vi "PID_controller_19.vi"() -> ()   [LabVIEW 2011]
panel:
  out "Angle (deg)":dbl format="%.1f"
  in  "Local":bool
  in  "Hold":bool
  out "tune_Method":u16(ring) items=["Setpoint", "Angle"]
  in  "Method":u16(ring)=1 items=["Setpoint", "Angle"]
  in  "Setpoint":u16(ring)=2 items=["A", "B", "C", "D"]
  out "do_tune":bool
  in  "Tune":bool
  out "Tune Set Point (torr)":dbl format="%.2f"
  in  "stop":bool
  out "fit":cluster{"element":dbl, "Value":dbl}[](array[cluster])
  out "err_avg":dbl
  out "Setpoint":string
  in  "Ks":dbl
  out "dt(s)":dbl
  out "windup error":dbl
  out "tPrev":dbl
  out "target value":dbl
  out "error(t-t0)":cluster{dbl, "Value":dbl}[](array[cluster])
  out "error":dbl
  out "tStart(s)":dbl
  out "S00":dbl
  out "S10":dbl
  out "S20":dbl
  out "S11":dbl
  out "S01":dbl
  out "weight":dbl[](array[numeric])
  in  "# of points to watch":i32=60
  in  "tSmooth(s)":dbl=4.0
  out "t0":dbl
  out "error(t)":cluster{dbl, "Value":dbl}[](array[cluster])
  out "IO error":errorcluster
  out "first":bool=TRUE
  out "XY Graph":T1(graph)
  out "current value":dbl
  in  "Period (s)":dbl=1.0
  out "dValue":dbl
  out "derivative":dbl
  out "integral":dbl
  in  "Angle (deg)":dbl format="%.1f"
  in  "Kd":dbl=0.4
  in  "Ki":dbl
  in  "Kp":dbl=0.1
  out "P (torr)":dbl format="%.2f"
  in  "Set Point (torr)":dbl format="%.2f"
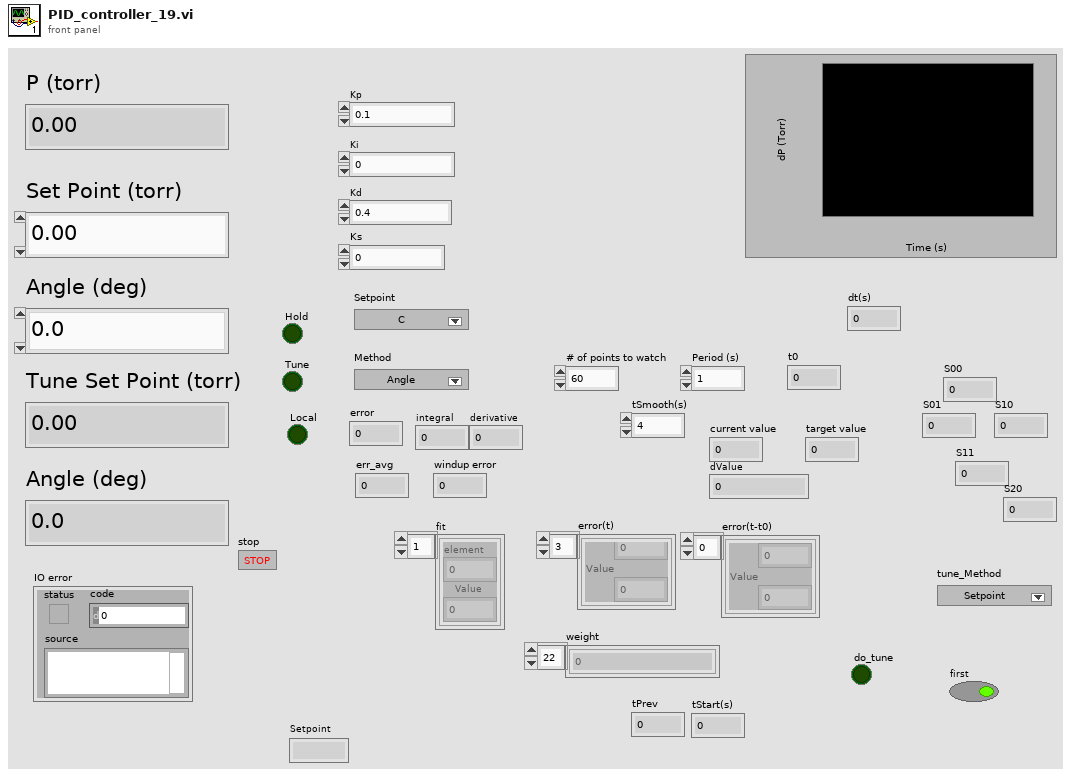
[diagram p1: front panel]
types:
  T1 = cluster{"Value":cluster{"element":dbl, "Value":dbl}[]}[]
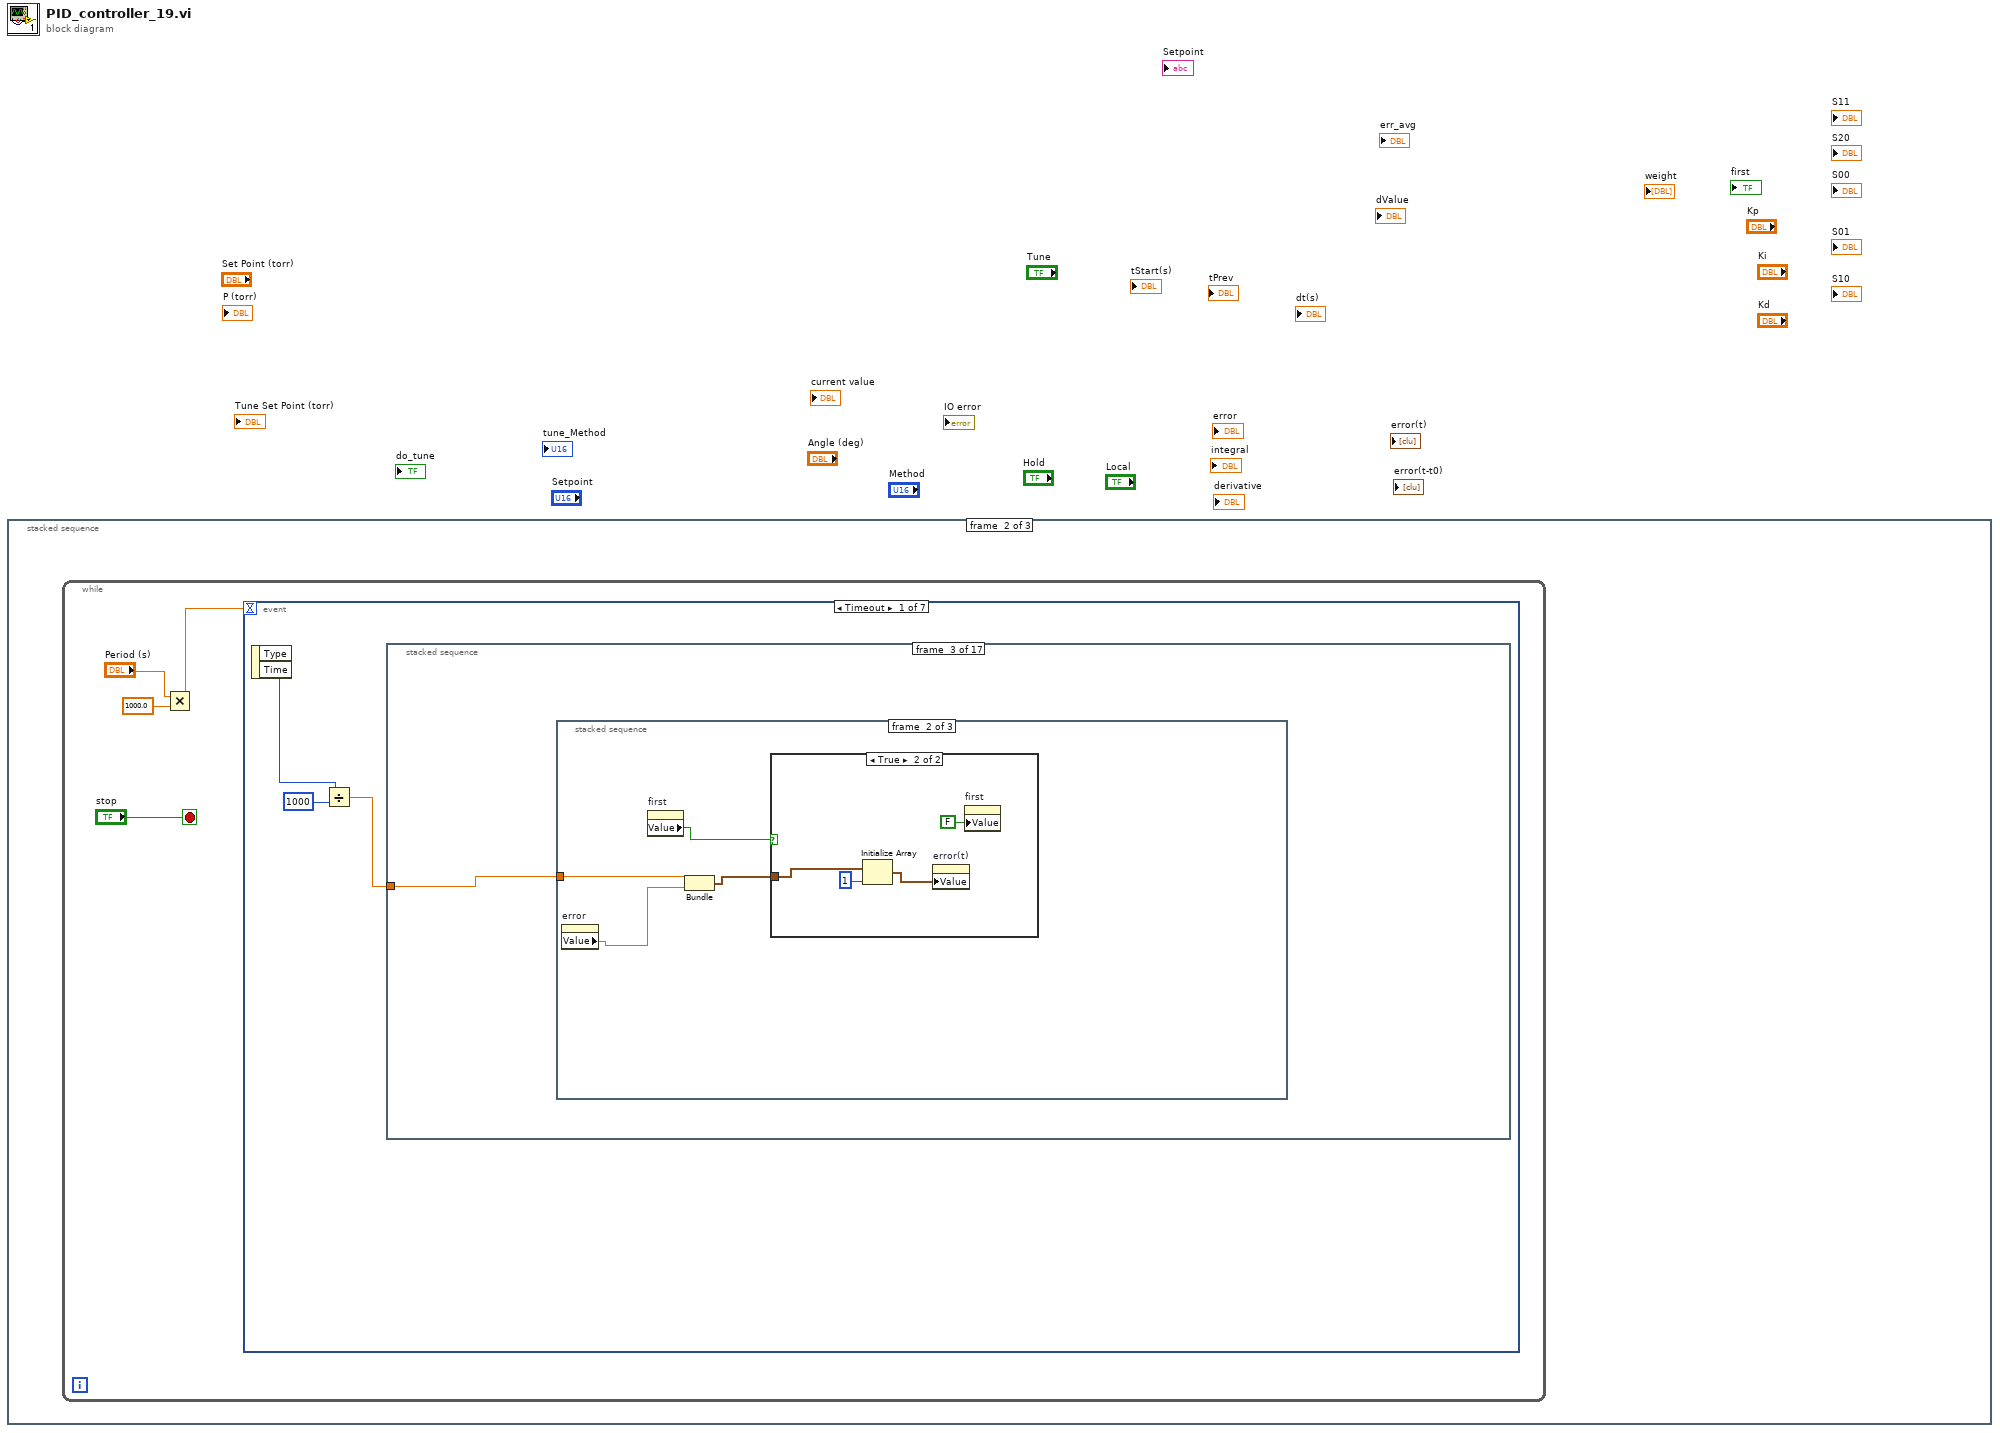
[diagram p0: block diagram]
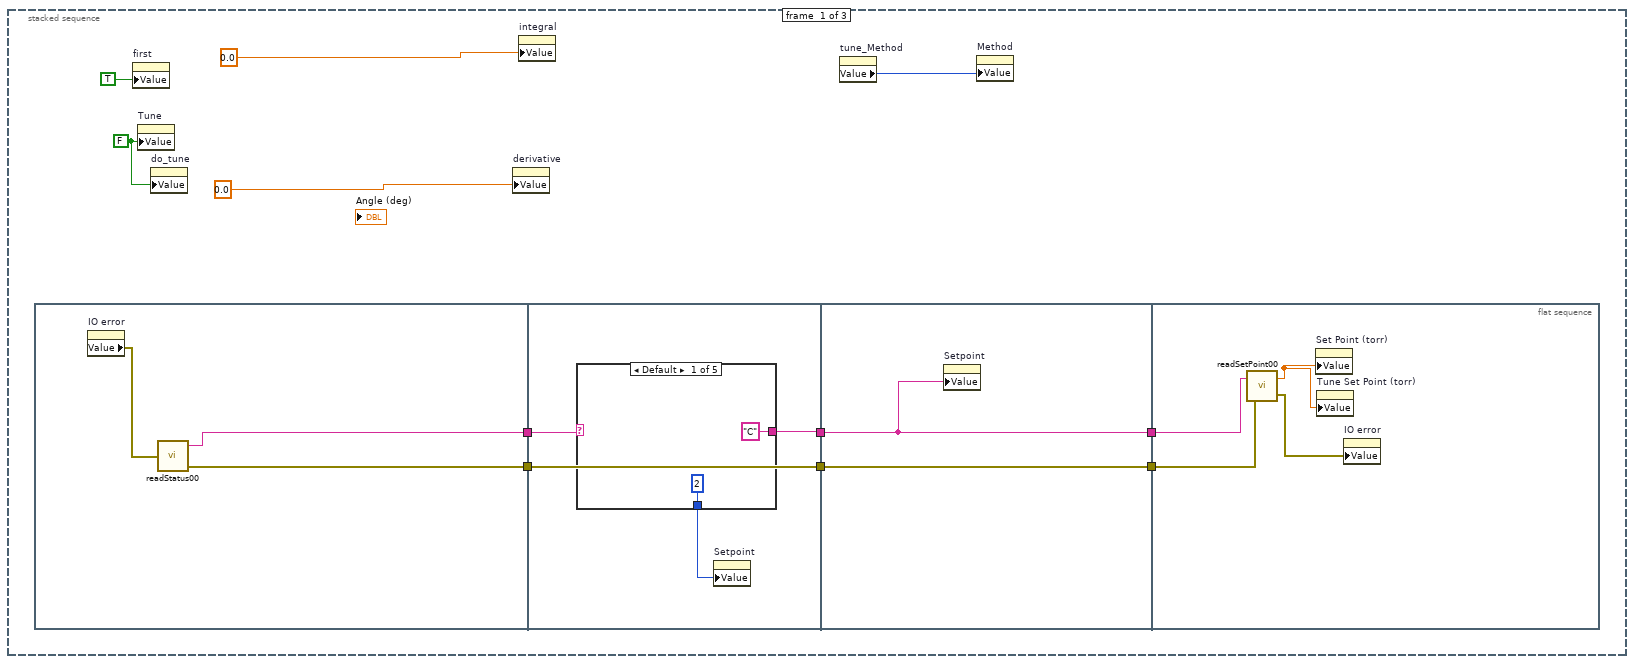
[diagram p2: hidden frame]
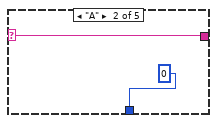
[diagram p3: hidden frame]
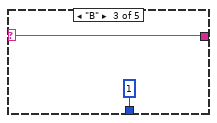
[diagram p4: hidden frame]
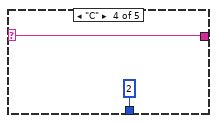
[diagram p5: hidden frame]
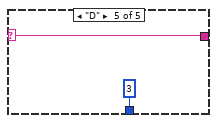
[diagram p6: hidden frame]
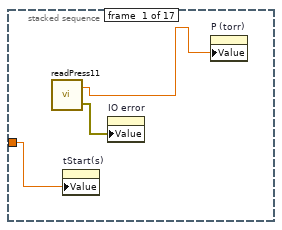
[diagram p7: hidden frame]
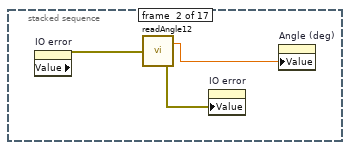
[diagram p8: hidden frame]
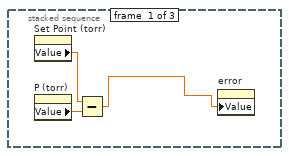
[diagram p9: hidden frame]
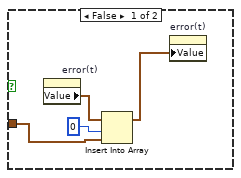
[diagram p10: hidden frame]
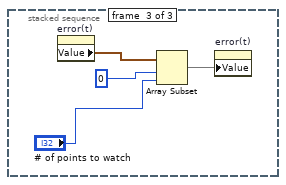
[diagram p11: hidden frame]
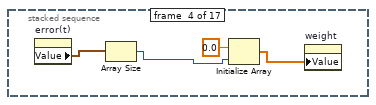
[diagram p12: hidden frame]
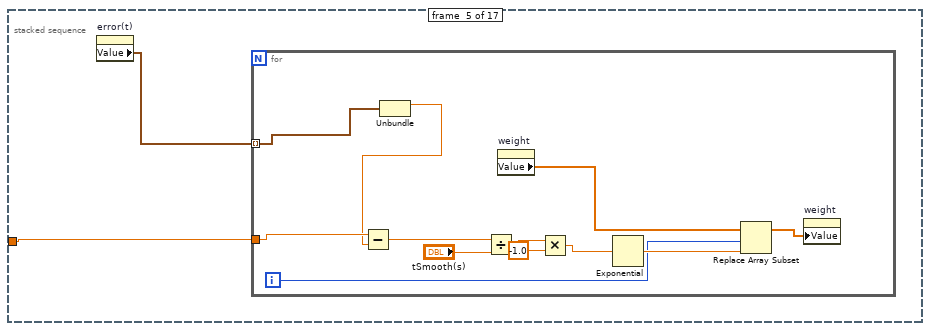
[diagram p13: hidden frame]
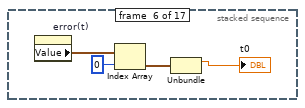
[diagram p14: hidden frame]
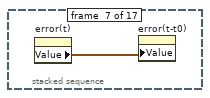
[diagram p15: hidden frame]
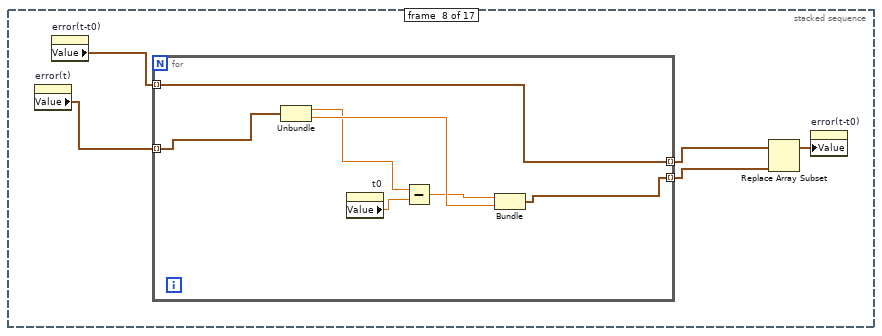
[diagram p16: hidden frame]
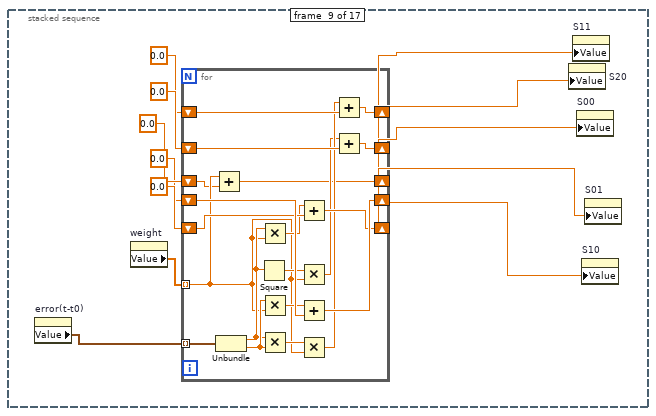
[diagram p17: hidden frame]
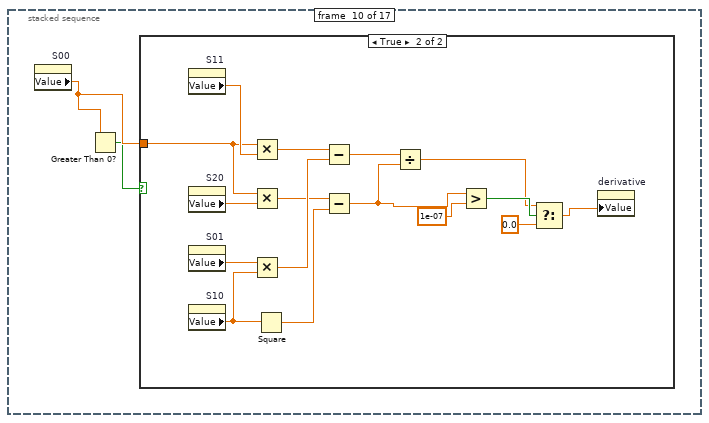
[diagram p18: hidden frame]
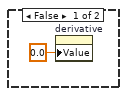
[diagram p19: hidden frame]
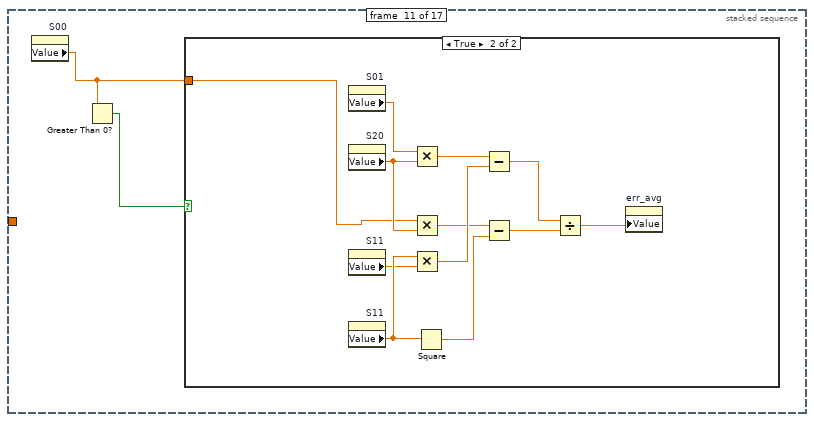
[diagram p20: hidden frame]
diagram:
  n1 = stacked-sequence {
    frame #0 {
      w8 = FALSE ("Tune")
      n2 = flat-sequence {
        tunnel: [w13] -> w7
        tunnel: [w12] -> w6
        tunnel: w7 -> [w17]
        tunnel: [w16] -> w5
        tunnel: w6 -> [w18]
        tunnel: [w18] -> w3
        tunnel: w5 -> [w29]
        tunnel: [w29] -> w4
        tunnel: w3 -> [w30]
        tunnel: [w30] -> w2
        tunnel: w4 -> [w34]
        tunnel: w2 -> [w33]
        frame #0 {
          n3 = property on="IO error" class="Clust (strict)"() -> ("Value"=w14:errorcluster)  [unwired: 2 in, 2 out]
          n4 = call "readStatus00.vi"("error in"=w14) -> ("Setpoint"=w13:string, "error out"=w12:errorcluster)  [unwired: 1 out]
        }
        frame #1 {
          n5 = case shown="Default" w17 {
            selector: w17 -> [_ w22 w23 w25 w27]
            tunnel: ["C" w22 w23 w25 w27] -> w16
            tunnel: [u16 2 ("Ring") u16 0 ("Ring") u16 1 ("Ring") u16 2 ("Ring") u16 3 ("Ring")] -> w15
            frame Default {
            }
            frame "A" {
            }
            frame "B" {
            }
            frame "C" {
            }
            frame "D" {
            }
          }
          n6 = property on="Setpoint" class="Ring (strict)"("Value"=w15) -> ()  [unwired: 2 in, 2 out]
        }
        frame #2 {
          n7 = property on="Setpoint" class="Str"("Value"=w29) -> ()  [unwired: 2 in, 2 out]
        }
        frame #3 {
          n8 = call "readSetPoint00.vi"("error in"=w33, "Setpoint"=w34) -> ("error out"=w32:errorcluster, "P"=w31:dbl)
          n9 = property on="Set Point (torr)" class="DigNum (strict)"("Value"=w31) -> ()  [unwired: 2 in, 2 out]
          n10 = property on="Tune Set Point (torr)" class="DigNum (strict)"("Value"=w31) -> ()  [unwired: 2 in, 2 out]
          n11 = property on="IO error" class="Clust (strict)"("Value"=w32) -> ()  [unwired: 2 in, 2 out]
        }
      }
      n12 = property on="first" class="Bool (strict)"("Value"=TRUE ("first")) -> ()  [unwired: 2 in, 2 out]
      n13 = property on="Tune" class="Bool (strict)"("Value"=w8) -> ()  [unwired: 2 in, 2 out]
      n14 = property on="do_tune" class="Bool (strict)"("Value"=w8) -> ()  [unwired: 2 in, 2 out]
      n15 = property on="derivative" class="DigNum (strict)"("Value"=0.0 ("derivative")) -> ()  [unwired: 2 in, 2 out]
      n16 = property on="integral" class="DigNum (strict)"("Value"=0.0 ("integral")) -> ()  [unwired: 2 in, 2 out]
      n17 = property on="tune_Method" class="Ring (strict)"() -> ("Value"=w1:u16)  [unwired: 2 in, 2 out]
      n18 = property on="Method" class="Ring (strict)"("Value"=w1) -> ()  [unwired: 2 in, 2 out]
    }
    frame #1 {
      n19 = while {
        stop <- "stop" stop-if-true
        n20 = Multiply(x="Period (s)", y=1000.0) -> (x*y=w36:dbl)
        n21 = event shown="[0] Timeout" {
          selector: _ -> [_ _ _ _ _ _ _]
          dyn-events: _ -> [_ _ _ _ _ _ _]
          timeout: w36 -> [_ _ _ _ _ _ _]
          event Timeout {
            n22 = event-data() -> ("Time"=w41:u32)  [unwired: 1 in, 1 out]
            n23 = Divide(x=w41, y=u32 1000) -> (x/y=w39:dbl)
            n24 = stacked-sequence {
              tunnel: w39 -> [w42 _ w48 _ w72 _ _ _ _ _ _ _ _ _ _ _ _]
              frame #0 {
                n25 = call "readPress11.vi"() -> ("P"=w44:dbl, "error out"=w43:errorcluster)  [unwired: 1 in]
                n26 = property on="tStart(s)" class="DigNum (strict)"("Value"=w42) -> ()  [unwired: 2 in, 2 out]
                n27 = property on="IO error" class="Clust (strict)"("Value"=w43) -> ()  [unwired: 2 in, 2 out]
                n28 = property on="P (torr)" class="DigNum (strict)"("Value"=w44) -> ()  [unwired: 2 in, 2 out]
              }
              frame #1 {
                n29 = property on="IO error" class="Clust (strict)"() -> ("Value"=w46:errorcluster)  [unwired: 2 in, 2 out]
                n30 = call "readAngle12.vi"("error in"=w46) -> ("angle"=w47:dbl, "error out"=w45:errorcluster)
                n31 = property on="IO error" class="Clust (strict)"("Value"=w45) -> ()  [unwired: 2 in, 2 out]
                n32 = property on="Angle (deg)" class="DigNum (strict)"("Value"=w47) -> ()  [unwired: 2 in, 2 out]
              }
              frame #2 {
                n33 = stacked-sequence {
                  tunnel: w48 -> [_ w54 _]
                  frame #0 {
                    n34 = property on="Set Point (torr)" class="DigNum (strict)"() -> ("Value"=w50:dbl)  [unwired: 2 in, 2 out]
                    n35 = property on="P (torr)" class="DigNum (strict)"() -> ("Value"=w51:dbl)  [unwired: 2 in, 2 out]
                    n36 = Subtract(x=w50, y=w51) -> (x-y=w49:dbl)
                    n37 = property on="error" class="DigNum (strict)"("Value"=w49) -> ()  [unwired: 2 in, 2 out]
                  }
                  frame #1 {
                    n38 = property on="error" class="DigNum (strict)"() -> ("Value"=w52:dbl)  [unwired: 2 in, 2 out]
                    n39 = property on="first" class="Bool (strict)"() -> ("Value"=w55:bool)  [unwired: 2 in, 2 out]
                    n40 = Bundle(w54, "Value"=w52) -> (w53:cluster{dbl, "Value":dbl})  [unwired: 1 in]
                    n41 = case shown="True" w55 {
                      tunnel: w53 -> [w57 w62]
                      frame False {
                        n42 = property on="error(t)" class="Arr (strict)"() -> ("Value"=w58:cluster{dbl, "Value":dbl}[])  [unwired: 2 in, 2 out]
                        n43 = Insert Into Array(array=w58, index=0, new element=w57) -> (w56:cluster{dbl, "Value":dbl}[])
                        n44 = property on="error(t)" class="Arr (strict)"("Value"=w56) -> ()  [unwired: 2 in, 2 out]
                      }
                      frame True {
                        n45 = Initialize Array(w62, 1 ("dimension size")) -> (w60:cluster{dbl, "Value":dbl}[])
                        n46 = property on="error(t)" class="Arr (strict)"("Value"=w60) -> ()  [unwired: 2 in, 2 out]
                        n47 = property on="first" class="Bool (strict)"("Value"=FALSE ("first")) -> ()  [unwired: 2 in, 2 out]
                      }
                    }
                  }
                  frame #2 {
                    n48 = property on="error(t)" class="Arr (strict)"() -> ("Value"=w65:cluster{dbl, "Value":dbl}[])  [unwired: 2 in, 2 out]
                    n49 = Array Subset(array=w65, index=0, length="# of points to watch") -> (w67:cluster{dbl, "Value":dbl}[])
                    n50 = property on="error(t)" class="Arr (strict)"("Value"=w67) -> ()  [unwired: 2 in, 2 out]
                  }
                }
              }
              frame #3 {
                n51 = property on="error(t)" class="Arr (strict)"() -> ("Value"=w68:cluster{dbl, "Value":dbl}[])  [unwired: 2 in, 2 out]
                n52 = Array Size(array=w68) -> (size(s)=w70:i32)
                n53 = Initialize Array(0.0 ("element"), w70) -> (w71:dbl[])
                n54 = property on="weight" class="Arr (strict)"("Value"=w71) -> ()  [unwired: 2 in, 2 out]
              }
              frame #4 {
                n55 = property on="error(t)" class="Arr (strict)"() -> ("Value"=w73:cluster{dbl, "Value":dbl}[])  [unwired: 2 in, 2 out]
                n56 = for {
                  tunnel: w73 -> [w85] mode=indexing
                  tunnel: w72 -> [w84]
                  i -> [w80]
                  n57 = Unbundle(w85) -> (w83:dbl)  [unwired: 1 out]
                  n58 = Subtract(x=w84, y=w83) -> (x-y=w78:dbl)
                  n59 = Divide(x=w78, y="tSmooth(s)") -> (x/y=w76:dbl)
                  n60 = property on="weight" class="Arr (strict)"() -> ("Value"=w81:dbl[])  [unwired: 2 in, 2 out]
                  n61 = Multiply(x=w76, y=-1.0) -> (x*y=w74:dbl)
                  n62 = Exponential(1:w74) -> (0:w82:dbl)
                  n63 = Replace Array Subset(array=w81, new element=w82, index=w80) -> (w79:dbl[])
                  n64 = property on="weight" class="Arr (strict)"("Value"=w79) -> ()  [unwired: 2 in, 2 out]
                }
              }
              frame #5 {
                n65 = property on="error(t)" class="Arr (strict)"() -> ("Value"=w86:cluster{dbl, "Value":dbl}[])  [unwired: 2 in, 2 out]
                n66 = Index Array(array=w86, index=0) -> (element=w88:cluster{dbl, "Value":dbl})
                n67 = Unbundle(w88) -> (→"t0":dbl)  [unwired: 1 out]
              }
              frame #6 {
                n68 = property on="error(t)" class="Arr (strict)"() -> ("Value"=w90:cluster{dbl, "Value":dbl}[])  [unwired: 2 in, 2 out]
                n69 = property on="error(t-t0)" class="Arr (strict)"("Value"=w90) -> ()  [unwired: 2 in, 2 out]
              }
              frame #7 {
                n70 = property on="error(t)" class="Arr (strict)"() -> ("Value"=w91:cluster{dbl, "Value":dbl}[])  [unwired: 2 in, 2 out]
                n71 = property on="error(t-t0)" class="Arr (strict)"() -> ("Value"=w93:cluster{dbl, "Value":dbl}[])  [unwired: 2 in, 2 out]
                n72 = for {
                  tunnel: w91 -> [w98] mode=indexing
                  tunnel: [w97] -> w92 mode=indexing
                  tunnel: w93 -> [w96] mode=indexing
                  tunnel: [w96] -> w94 mode=indexing
                  n73 = Unbundle(w98) -> (w99:dbl, "Value"=w101:dbl)
                  n74 = property on="t0" class="DigNum (strict)"() -> ("Value"=w102:dbl)  [unwired: 2 in, 2 out]
                  n75 = Subtract(x=w99, y=w102) -> (x-y=w100:dbl)
                  n76 = Bundle(w100, "Value"=w101) -> (w97:cluster{dbl, "Value":dbl})  [unwired: 1 in]
                }
                n77 = Replace Array Subset(array=w94, new element=w92) -> (w95:cluster{dbl, "Value":dbl}[])  [unwired: 1 in]
                n78 = property on="error(t-t0)" class="Arr (strict)"("Value"=w95) -> ()  [unwired: 2 in, 2 out]
              }
              frame #8 {
                n79 = property on="error(t-t0)" class="Arr (strict)"() -> ("Value"=w114:cluster{dbl, "Value":dbl}[])  [unwired: 2 in, 2 out]
                n80 = property on="weight" class="Arr (strict)"() -> ("Value"=w107:dbl[])  [unwired: 2 in, 2 out]
                n81 = for {
                  tunnel: w114 -> [w130] mode=indexing
                  shift-right: [w131] -> w112
                  shift-left: 0.0 -> [w134]
                  shift-right: [w127] -> w109
                  shift-left: 0.0 -> [w133]
                  shift-right: [w126] -> w110
                  shift-left: 0.0 -> [w132]
                  shift-right: [w128] -> w113
                  shift-left: 0.0 -> [w129]
                  tunnel: w107 -> [w117] mode=indexing
                  shift-right: [w115] -> w111
                  shift-left: 0.0 -> [w116]
                  n82 = Add(x=w117, y=w116) -> (x+y=w115:dbl)
                  n83 = Unbundle(w130) -> (w119:dbl, "Value"=w125:dbl)
                  n84 = Square(x=w119) -> (x^2=w121:dbl)
                  n85 = Multiply(x=w119, y=w117) -> (x*y=w118:dbl)
                  n86 = Multiply(x=w125, y=w117) -> (x*y=w124:dbl)
                  n87 = Multiply(x=w119, y=w125) -> (x*y=w123:dbl)
                  n88 = Add(x=w118, y=w129) -> (x+y=w128:dbl)
                  n89 = Multiply(x=w121, y=w117) -> (x*y=w120:dbl)
                  n90 = Add(x=w124, y=w134) -> (x+y=w131:dbl)
                  n91 = Multiply(x=w123, y=w117) -> (x*y=w122:dbl)
                  n92 = Add(x=w122, y=w133) -> (x+y=w127:dbl)
                  n93 = Add(x=w120, y=w132) -> (x+y=w126:dbl)
                }
                n94 = property on="S20" class="DigNum (strict)"("Value"=w110) -> ()  [unwired: 2 in, 2 out]
                n95 = property on="S11" class="DigNum (strict)"("Value"=w109) -> ()  [unwired: 2 in, 2 out]
                n96 = property on="S00" class="DigNum (strict)"("Value"=w111) -> ()  [unwired: 2 in, 2 out]
                n97 = property on="S10" class="DigNum (strict)"("Value"=w113) -> ()  [unwired: 2 in, 2 out]
                n98 = property on="S01" class="DigNum (strict)"("Value"=w112) -> ()  [unwired: 2 in, 2 out]
              }
              frame #9 {
                n99 = property on="S00" class="DigNum (strict)"() -> ("Value"=w136:dbl)  [unwired: 2 in, 2 out]
                n100 = Greater Than 0?(x=w136) -> (x > 0?=w135:bool)
                n101 = case shown="True" w135 {
                  tunnel: w136 -> [_ w145]
                  frame False {
                    n102 = property on="derivative" class="DigNum (strict)"("Value"=0.0 ("derivative")) -> ()  [unwired: 2 in, 2 out]
                  }
                  frame True {
                    n103 = property on="S11" class="DigNum (strict)"() -> ("Value"=w147:dbl)  [unwired: 2 in, 2 out]
                    n104 = property on="S20" class="DigNum (strict)"() -> ("Value"=w146:dbl)  [unwired: 2 in, 2 out]
                    n105 = property on="S01" class="DigNum (strict)"() -> ("Value"=w144:dbl)  [unwired: 2 in, 2 out]
                    n106 = property on="S10" class="DigNum (strict)"() -> ("Value"=w148:dbl)  [unwired: 2 in, 2 out]
                    n107 = Multiply(x=w145, y=w147) -> (x*y=w153:dbl)
                    n108 = Multiply(x=w145, y=w146) -> (x*y=w151:dbl)
                    n109 = Multiply(x=w144, y=w148) -> (x*y=w152:dbl)
                    n110 = Square(x=w148) -> (x^2=w150:dbl)
                    n111 = Subtract(x=w153, y=w152) -> (x-y=w149:dbl)
                    n112 = Subtract(x=w151, y=w150) -> (x-y=w143:dbl)
                    n113 = Divide(x=w149, y=w143) -> (x/y=w139:dbl)
                    n114 = Greater?(x=w143, y=1e-07) -> (0:w141:bool)
                    n115 = Select(t=w139, s=w141, f=0.0) -> (s? t:f=w140:dbl)
                    n116 = property on="derivative" class="DigNum (strict)"("Value"=w140) -> ()  [unwired: 2 in, 2 out]
                  }
                }
              }
              frame #10 {
                n117 = property on="S00" class="DigNum (strict)"() -> ("Value"=w155:dbl)  [unwired: 2 in, 2 out]
                n118 = Greater Than 0?(x=w155) -> (x > 0?=w154:bool)
                n119 = case shown="True" w154 {
                  tunnel: w155 -> [_ w158]
                  frame False {
                    n120 = property on="err_avg" class="DigNum (strict)"("Value"=0.0 ("Pavg")) -> ()  [unwired: 2 in, 2 out]
                  }
                  frame True {
                    n121 = property on="S01" class="DigNum (strict)"() -> ("Value"=w159:dbl)  [unwired: 2 in, 2 out]
                    n122 = property on="S20" class="DigNum (strict)"() -> ("Value"=w162:dbl)  [unwired: 2 in, 2 out]
                    n123 = property on="S11" class="DigNum (strict)"() -> ("Value"=w160:dbl)  [unwired: 2 in, 2 out]
                    n124 = property on="S11" class="DigNum (strict)"() -> ("Value"=w161:dbl)  [unwired: 2 in, 2 out]
                    n125 = Multiply(x=w159, y=w162) -> (x*y=w167:dbl)
                    n126 = Multiply(x=w158, y=w162) -> (x*y=w164:dbl)
                    n127 = Multiply(x=w161, y=w160) -> (x*y=w168:dbl)
                    n128 = Square(x=w161) -> (x^2=w165:dbl)
                    n129 = Subtract(x=w167, y=w168) -> (x-y=w163:dbl)
                    n130 = Subtract(x=w164, y=w165) -> (x-y=w166:dbl)
                    n131 = Divide(x=w163, y=w166) -> (x/y=w157:dbl)
                    n132 = property on="err_avg" class="DigNum (strict)"("Value"=w157) -> ()  [unwired: 2 in, 2 out]
                  }
                }
              }
              frame #11 {
                n133 = property on="error(t-t0)" class="Arr (strict)"() -> ("Value"=w169:cluster{dbl, "Value":dbl}[])  [unwired: 2 in, 2 out]
                n134 = Array Size(array=w169) -> (size(s)=w170:i32)
                n135 = Greater?(x=w170, y=1) -> (0:w172:bool)
                n136 = case shown="True" w172 {
                  frame False {
                  }
                  frame True {
                    n137 = property on="error(t-t0)" class="Arr (strict)"() -> ("Value"=w184:cluster{dbl, "Value":dbl}[])  [unwired: 2 in, 2 out]
                    n138 = Array Size(array=w184) -> (size(s)=w192:i32)
                    n139 = Index Array(array=w184, index=0) -> (element=w190:cluster{dbl, "Value":dbl})
                    n140 = property on="tSmooth(s)" class="DigNum (strict)"() -> ("Value"=w174:dbl)  [unwired: 2 in, 2 out]
                    n141 = Unbundle(w190) -> (w180:dbl)  [unwired: 1 out]
                    n142 = Decrement(x=w192) -> (x-1=w191:i32)
                    n143 = Index Array(array=w184, index=w191) -> (element=w189:cluster{dbl, "Value":dbl})
                    n144 = Multiply(x=w174, y=2.0) -> (x*y=w173:dbl)
                    n145 = Unbundle(w189) -> (w179:dbl)  [unwired: 1 out]
                    n146 = Subtract(x=w180, y=w173) -> (x-y=w177:dbl)
                    n147 = Greater?(x=w179, y=w177) -> (0:w178:bool)
                    n148 = property on="derivative" class="DigNum (strict)"() -> ("Value"=w188:dbl)  [unwired: 2 in, 2 out]
                    n149 = Select(t=w179, s=w178, f=w177) -> (s? t:f=w176:dbl)
                    n150 = property on="error" class="DigNum (strict)"() -> ("Value"=w186:dbl)  [unwired: 2 in, 2 out]
                    n151 = Multiply(x=w176, y=w188) -> (x*y=w187:dbl)
                    n152 = Add(x=w186, y=w187) -> (x+y=w185:dbl)
                    n153 = Bundle(w180, "Value"=w186) -> (w183:cluster{dbl, "Value":dbl})  [unwired: 1 in]
                    n154 = Bundle(w176, w185) -> (w182:cluster{dbl, dbl})  [unwired: 1 in]
                    n155 = Build Array(w183, w182) -> (→"fit":cluster{dbl, "Value":dbl}[])
                  }
                }
              }
              frame #12 {
                n156 = property on="error" class="DigNum (strict)"() -> ("Value"=w196:dbl)  [unwired: 2 in, 2 out]
                n157 = property on="tPrev" class="DigNum (strict)"() -> ("Value"=w195:dbl)  [unwired: 2 in, 2 out]
                n158 = property on="tStart(s)" class="DigNum (strict)"() -> ("Value"=w194:dbl)  [unwired: 2 in, 2 out]
                n159 = Subtract(x=w194, y=w195) -> (x-y=w200:dbl)
                n160 = property on="dt(s)" class="DigNum (strict)"("Value"=w200) -> ()  [unwired: 2 in, 2 out]
                n161 = property on="integral" class="DigNum (strict)"() -> ("Value"=w198:dbl)  [unwired: 2 in, 2 out]
                n162 = Multiply(x=w196, y=w200) -> (x*y=w197:dbl)
                n163 = Add(x=w197, y=w198) -> (x+y=w199:dbl)
                n164 = property on="integral" class="DigNum (strict)"("Value"=w199) -> ()  [unwired: 2 in, 2 out]
              }
              frame #13 {
                n165 = property on="error" class="DigNum (strict)"() -> ("Value"=w213:dbl)  [unwired: 2 in, 2 out]
                n166 = property on="tune_Method" class="Ring (strict)"() -> ("Value"=w203:u16)  [unwired: 2 in, 2 out]
                n167 = property on="Kp" class="DigNum (strict)"() -> ("Value"=w202:dbl)  [unwired: 2 in, 2 out]
                n168 = property on="integral" class="DigNum (strict)"() -> ("Value"=w205:dbl)  [unwired: 2 in, 2 out]
                n169 = property on="derivative" class="DigNum (strict)"() -> ("Value"=w207:dbl)  [unwired: 2 in, 2 out]
                n170 = property on="Ki" class="DigNum (strict)"() -> ("Value"=w204:dbl)  [unwired: 2 in, 2 out]
                n171 = property on="Kd" class="DigNum (strict)"() -> ("Value"=w206:dbl)  [unwired: 2 in, 2 out]
                n172 = case shown="0, Default" w203 {
                  tunnel: w202 -> [w214 w217]
                  tunnel: [w214 w215] -> w201
                  frame 0, Default {
                  }
                  frame 1 {
                    n173 = Multiply(x=w217, y=-1.0) -> (x*y=w215:dbl)
                  }
                }
                n174 = Multiply(x=w206, y=w207) -> (x*y=w210:dbl)
                n175 = Multiply(x=w204, y=w205) -> (x*y=w209:dbl)
                n176 = Multiply(x=w201, y=w213) -> (x*y=w208:dbl)
                n177 = Add(x=w208, y=w209) -> (x+y=w211:dbl)
                n178 = Add(x=w211, y=w210) -> (x+y=w212:dbl)
                n179 = property on="dValue" class="DigNum (strict)"("Value"=w212) -> ()  [unwired: 2 in, 2 out]
              }
              frame #14 {
                n180 = property on="do_tune" class="Bool (strict)"() -> ("Value"=w218:bool)  [unwired: 2 in, 2 out]
                n181 = case shown="True" w218 {
                  frame False {
                  }
                  frame True {
                    w231 = 90.0 ("y")
                    n182 = property on="dValue" class="DigNum (strict)"() -> ("Value"=w236:dbl)  [unwired: 2 in, 2 out]
                    n183 = property on="current value" class="DigNum (strict)"() -> ("Value"=w237:dbl)  [unwired: 2 in, 2 out]
                    n184 = Add(x=w237, y=w236) -> (x+y=w223:dbl)
                    "target value" <- w223
                    n185 = Less Than 0?(x=w223) -> (x < 0?=w235:bool)
                    n186 = Select(t=0.0, s=w235, f=w223) -> (s? t:f=w232:dbl)
                    n187 = property on="IO error" class="Clust (strict)"() -> ("Value"=w221:errorcluster)  [unwired: 2 in, 2 out]
                    n188 = Greater?(x=w232, y=w231) -> (0:w233:bool)
                    n189 = Select(t=w231, s=w233, f=w232) -> (s? t:f=w220:dbl)
                    n190 = Subtract(x=w220, y=w223) -> (x-y=w230:dbl)
                    "windup error" <- w230
                    n191 = property on="dt(s)" class="DigNum (strict)"() -> ("Value"=w229:dbl)  [unwired: 2 in, 2 out]
                    n192 = property on="current value" class="DigNum (strict)"("Value"=w220) -> ()  [unwired: 2 in, 2 out]
                    n193 = property on="tune_Method" class="Ring (strict)"() -> ("Value"=w222:u16)  [unwired: 2 in, 2 out]
                    n194 = Multiply(x=w230, y=w229) -> (x*y=w228:dbl)
                    n195 = property on="integral" class="DigNum (strict)"() -> ("Value"=w225:dbl)  [unwired: 2 in, 2 out]
                    n196 = Multiply(x="Ks", y=w228) -> (x*y=w226:dbl)
                    n197 = case shown="1" w222 {
                      tunnel: w221 -> [w241 w244]
                      tunnel: w220 -> [w240 w243]
                      tunnel: [w238 w242] -> w219
                      frame 0, Default {
                        n198 = property on="Setpoint" class="Str"() -> ("Value"=w239:string)  [unwired: 2 in, 2 out]
                        n199 = property on="Tune Set Point (torr)" class="DigNum (strict)"("Value"=w240) -> ()  [unwired: 2 in, 2 out]
                        n200 = call "writeSetPoint_00.vi"("error in"=w241, "P (Torr)"=w240, "Setpoint"=w239) -> ("error out"=w238:errorcluster)
                      }
                      frame 1 {
                        n201 = call "setAngle_00.vi"("error in (no error)"=w244, "Angle (deg)"=w243) -> ("error out"=w242:errorcluster)
                      }
                    }
                    n202 = Add(x=w226, y=w225) -> (x+y=w224:dbl)
                    n203 = property on="integral" class="DigNum (strict)"("Value"=w224) -> ()  [unwired: 2 in, 2 out]
                    n204 = property on="IO error" class="Clust (strict)"("Value"=w219) -> ()  [unwired: 2 in, 2 out]
                  }
                }
              }
              frame #15 {
                n205 = property on="fit" class="Arr (strict)"() -> ("Value"=w247:cluster{"element":dbl, "Value":dbl}[])  [unwired: 2 in, 2 out]
                n206 = property on="error(t-t0)" class="Arr (strict)"() -> ("Value"=w246:cluster{dbl, "Value":dbl}[])  [unwired: 2 in, 2 out]
                n207 = Build Cluster Array(w246, w247) -> (→"XY Graph":T1)
              }
              frame #16 {
                n208 = property on="tStart(s)" class="DigNum (strict)"() -> ("Value"=w248:dbl)  [unwired: 2 in, 2 out]
                n209 = property on="tPrev" class="DigNum (strict)"("Value"=w248) -> ()  [unwired: 2 in, 2 out]
              }
            }
          }
          event "Hold": Value Change {
            n210 = event-data() -> ()  [unwired: 1 in, 5 out]
            n211 = property on="Hold" class="Bool (strict)"() -> ("Value"=w249:bool)  [unwired: 2 in, 2 out]
            n212 = case shown="False" w249 {
              frame False {
                n213 = property on="Local" class="Bool (strict)"() -> ("Value"=w250:bool)  [unwired: 2 in, 2 out]
                n214 = case shown="False" w250 {
                  frame False {
                    n215 = property on="IO error" class="Clust (strict)"() -> ("Value"=w254:errorcluster)  [unwired: 2 in, 2 out]
                    n216 = property on="Setpoint" class="Str"() -> ("Value"=w251:string)  [unwired: 2 in, 2 out]
                    n217 = call "readSetPoint00.vi"("error in"=w254, "Setpoint"=w251) -> ("error out"=w253:errorcluster, "P"=w252:dbl)
                    n218 = property on="Tune Set Point (torr)" class="DigNum (strict)"("Value"=w252) -> ()  [unwired: 2 in, 2 out]
                    n219 = property on="Set Point (torr)" class="DigNum (strict)"("Value"=w252) -> ()  [unwired: 2 in, 2 out]
                    n220 = property on="IO error" class="Clust (strict)"("Value"=w253) -> ()  [unwired: 2 in, 2 out]
                  }
                  frame True {
                  }
                }
              }
              frame True {
                n221 = property on="IO error" class="Clust (strict)"() -> ("Value"=w258:errorcluster)  [unwired: 2 in, 2 out]
                n222 = property on="Tune" class="Bool (strict)"("Value"=FALSE ("Tune")) -> ()  [unwired: 2 in, 2 out]
                n223 = property on="Local" class="Bool (strict)"("Value"=FALSE ("Local")) -> ()  [unwired: 2 in, 2 out]
                n224 = call "WriteAdaptorr03.vi"("error in (no error)"=w258, "string to write"="H") -> ("error out"=w257:errorcluster)
                n225 = property on="IO error" class="Clust (strict)"("Value"=w257) -> ()  [unwired: 2 in, 2 out]
              }
            }
          }
          event "Local": Value Change {
            n226 = event-data() -> ()  [unwired: 1 in, 5 out]
            n227 = property on="Local" class="Bool (strict)"() -> ("Value"=w260:bool)  [unwired: 2 in, 2 out]
            n228 = case shown="True" w260 {
              frame False {
                n229 = property on="IO error" class="Clust (strict)"() -> ("Value"=w263:errorcluster)  [unwired: 2 in, 2 out]
                n230 = call "WriteAdaptorr03.vi"("error in (no error)"=w263, "string to write"="H") -> ("error out"=w262:errorcluster)
                n231 = property on="Hold" class="Bool (strict)"("Value"=TRUE ("Hold")) -> ()  [unwired: 2 in, 2 out]
                n232 = property on="IO error" class="Clust (strict)"("Value"=w262) -> ()  [unwired: 2 in, 2 out]
              }
              frame True {
                n233 = property on="IO error" class="Clust (strict)"() -> ("Value"=w267:errorcluster)  [unwired: 2 in, 2 out]
                n234 = call "WriteAdaptorr03.vi"("error in (no error)"=w267, "string to write"="D5") -> ("error out"=w268:errorcluster)
                n235 = property on="Hold" class="Bool (strict)"("Value"=FALSE ("Hold")) -> ()  [unwired: 2 in, 2 out]
                n236 = property on="IO error" class="Clust (strict)"("Value"=w268) -> ()  [unwired: 2 in, 2 out]
              }
            }
          }
          event "Tune": Value Change {
            n237 = event-data() -> ()  [unwired: 1 in, 5 out]
            n238 = property on="Tune" class="Bool (strict)"() -> ("Value"=w269:bool)  [unwired: 2 in, 2 out]
            n239 = property on="do_tune" class="Bool (strict)"("Value"=w269) -> ()  [unwired: 2 in, 2 out]
            n240 = case shown="True" w269 {
              frame False {
                n241 = property on="tune_Method" class="Ring (strict)"() -> ("Value"=w270:u16)  [unwired: 2 in, 2 out]
                n242 = case shown="1" w270 {
                  frame 0, Default {
                    n243 = property on="Set Point (torr)" class="DigNum (strict)"() -> ("Value"=w273:dbl)  [unwired: 2 in, 2 out]
                    n244 = property on="Setpoint" class="Str"() -> ("Value"=w274:string)  [unwired: 2 in, 2 out]
                    n245 = property on="IO error" class="Clust (strict)"() -> ("Value"=w272:errorcluster)  [unwired: 2 in, 2 out]
                    n246 = call "writeSetPoint_00.vi"("error in"=w272, "P (Torr)"=w273, "Setpoint"=w274) -> ("error out"=w271:errorcluster)
                    n247 = property on="IO error" class="Clust (strict)"("Value"=w271) -> ()  [unwired: 2 in, 2 out]
                  }
                  frame 1 {
                    n248 = flat-sequence {
                      frame #0 {
                        n249 = call "WriteAdaptorr03.vi"("string to write"="D5") -> ()  [unwired: 1 in, 1 out]
                      }
                      frame #1 {
                        n250 = property on="Setpoint" class="Str"() -> ("Value"=w277:string)  [unwired: 2 in, 2 out]
                        n251 = Concatenate Strings("Press ", w277, " on AdapTorr") -> (w276:string)
                        n252 = One Button Dialog(message=w276) -> ()  [unwired: 1 in, 1 out]
                      }
                    }
                  }
                }
              }
              frame True {
                n253 = property on="tune_Method" class="Ring (strict)"() -> ("Value"=w281:u16)  [unwired: 2 in, 2 out]
                n254 = case shown="0, Default" w281 {
                  frame 0, Default {
                    n255 = property on="IO error" class="Clust (strict)"() -> ("Value"=w284:errorcluster)  [unwired: 2 in, 2 out]
                    n256 = property on="Setpoint" class="Str"() -> ("Value"=w283:string)  [unwired: 2 in, 2 out]
                    n257 = call "readSetPoint00.vi"("error in"=w284, "Setpoint"=w283) -> ("error out"=w285:errorcluster, "P"=w282:dbl)
                    n258 = property on="Tune Set Point (torr)" class="DigNum (strict)"("Value"=w282) -> ()  [unwired: 2 in, 2 out]
                    n259 = property on="Set Point (torr)" class="DigNum (strict)"("Value"=w282) -> ()  [unwired: 2 in, 2 out]
                    n260 = property on="IO error" class="Clust (strict)"("Value"=w285) -> ()  [unwired: 2 in, 2 out]
                    n261 = property on="current value" class="DigNum (strict)"("Value"=w282) -> ()  [unwired: 2 in, 2 out]
                  }
                  frame 1 {
                    n262 = property on="Angle (deg)" class="DigNum (strict)"() -> ("Value"=w286:dbl)  [unwired: 2 in, 2 out]
                    n263 = property on="current value" class="DigNum (strict)"("Value"=w286) -> ()  [unwired: 2 in, 2 out]
                  }
                }
                n264 = property on="integral" class="DigNum (strict)"("Value"=0.0 ("integral")) -> ()  [unwired: 2 in, 2 out]
              }
            }
          }
          event "Set Point (torr)": Value Change {
            n265 = event-data() -> ()  [unwired: 1 in, 5 out]
            n266 = property on="Set Point (torr)" class="DigNum (strict)"() -> ("Value"=w289:dbl)  [unwired: 2 in, 2 out]
            n267 = property on="Setpoint" class="Str"() -> ("Value"=w290:string)  [unwired: 2 in, 2 out]
            n268 = property on="IO error" class="Clust (strict)"() -> ("Value"=w288:errorcluster)  [unwired: 2 in, 2 out]
            n269 = call "writeSetPoint_00.vi"("error in"=w288, "P (Torr)"=w289, "Setpoint"=w290) -> ("error out"=w287:errorcluster)
            n270 = property on="IO error" class="Clust (strict)"("Value"=w287) -> ()  [unwired: 2 in, 2 out]
          }
          event "Setpoint": Value Change {
            n271 = event-data() -> ()  [unwired: 1 in, 5 out]
            n272 = property on="Setpoint" class="Ring (strict)"() -> ("Value"=w295:u16)  [unwired: 2 in, 2 out]
            n273 = case shown="3" w295 {
              tunnel: ["A" "B" "C" "D"] -> w291
              frame 0, Default {
              }
              frame 1 {
              }
              frame 2 {
              }
              frame 3 {
              }
            }
            n274 = property on="Setpoint" class="Str"("Value"=w291) -> ()  [unwired: 2 in, 2 out]
            n275 = property on="IO error" class="Clust (strict)"() -> ("Value"=w292:errorcluster)  [unwired: 2 in, 2 out]
            n276 = call "readSetPoint00.vi"("error in"=w292, "Setpoint"=w291) -> ("error out"=w293:errorcluster, "P"=w294:dbl)
            n277 = property on="Set Point (torr)" class="DigNum (strict)"("Value"=w294) -> ()  [unwired: 2 in, 2 out]
            n278 = property on="Tune Set Point (torr)" class="DigNum (strict)"("Value"=w294) -> ()  [unwired: 2 in, 2 out]
            n279 = property on="IO error" class="Clust (strict)"("Value"=w293) -> ()  [unwired: 2 in, 2 out]
          }
          event "Method": Value Change {
            n280 = event-data() -> ()  [unwired: 1 in, 5 out]
            n281 = property on="Method" class="Ring (strict)"() -> ("Value"=w300:u16)  [unwired: 2 in, 2 out]
            n282 = case shown="1" w300 {
              frame 0, Default {
              }
              frame 1 {
                n283 = property on="do_tune" class="Bool (strict)"() -> ("Value"=w301:bool)  [unwired: 2 in, 2 out]
                n284 = case shown="True" w301 {
                  frame False {
                  }
                  frame True {
                    n285 = flat-sequence {
                      frame #0 {
                        n286 = call "WriteAdaptorr03.vi"("string to write"="D5") -> ()  [unwired: 1 in, 1 out]
                      }
                      frame #1 {
                        n287 = property on="Setpoint" class="Str"() -> ("Value"=w304:string)  [unwired: 2 in, 2 out]
                        n288 = Concatenate Strings("Press ", w304, " on AdapTorr") -> (w303:string)
                        n289 = One Button Dialog(message=w303) -> ()  [unwired: 1 in, 1 out]
                      }
                    }
                  }
                }
              }
            }
            n290 = property on="tune_Method" class="Ring (strict)"("Value"=w300) -> ()  [unwired: 2 in, 2 out]
          }
        }
      }
    }
    frame #2 {
      n291 = property on="tune_Method" class="Ring (strict)"() -> ("Value"=w307:u16)  [unwired: 2 in, 2 out]
      n292 = case shown="1" w307 {
        frame 0, Default {
        }
        frame 1 {
          n293 = flat-sequence {
            frame #0 {
              n294 = property on="IO error" class="Clust (strict)"() -> ("Value"=w309:errorcluster)  [unwired: 2 in, 2 out]
              n295 = call "setLocal_And_Hold_00.vi"("error in (no error)"=w309) -> ("error out"=w308:errorcluster)
              n296 = property on="IO error" class="Clust (strict)"("Value"=w308) -> ()  [unwired: 2 in, 2 out]
            }
            frame #1 {
              n297 = property on="Setpoint" class="Str"() -> ("Value"=w311:string)  [unwired: 2 in, 2 out]
              n298 = Concatenate Strings("Press ", w311, " on AdapTorr") -> (w310:string)
              n299 = One Button Dialog(message=w310) -> ()  [unwired: 1 in, 1 out]
            }
          }
        }
      }
    }
  }
